vi "forceOutputState.vi"(8 "error in (no error)":errorcluster, 9 "calibratedValues":dbl[](array[numeric]), 10 "channel_addresses":string[](array[string]), 11 "niDAQmxAO in":refnum<class "niDAQmxAO.lvclass">) -> (0 "error out":errorcluster, 3 "niDAQmxAO out":refnum<class "niDAQmxAO.lvclass">)   [LabVIEW 2011, in "Hardware.lvlib" / "Channels.lvlib" / "niDAQmxAO.lvclass"]
uses:
  niDAQmxAO.lvclass
  <vilib>/DAQmx/write.llb/DAQmx Write (Analog DBL 1Chan 1Samp).vi
  <vilib>/DAQmx/write.llb/DAQmx Write (Analog 1D DBL NChan 1Samp).vi
  <vilib>/DAQmx/create/channels.llb/DAQmx Create Channel (AO-Voltage-Basic).vi
  <vilib>/DAQmx/miscellaneous.llb/DAQmx Fill In Error Info.vi
  AnalogOutput.lvclass
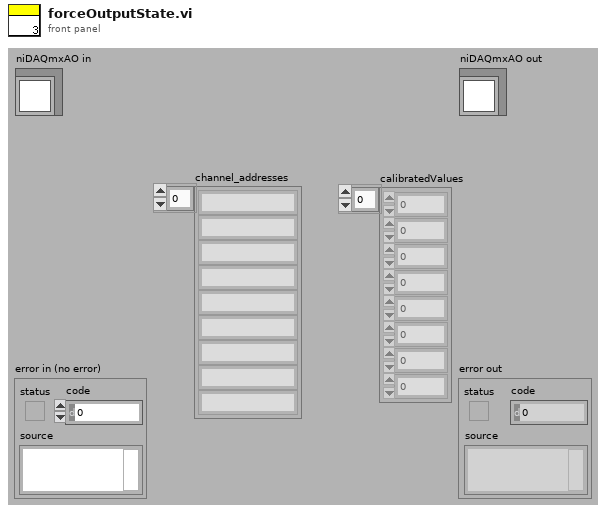
[diagram p1: front panel]
types:
  T1 = cluster{"channel_addresses":string[], "calibratedValues":dbl[]}
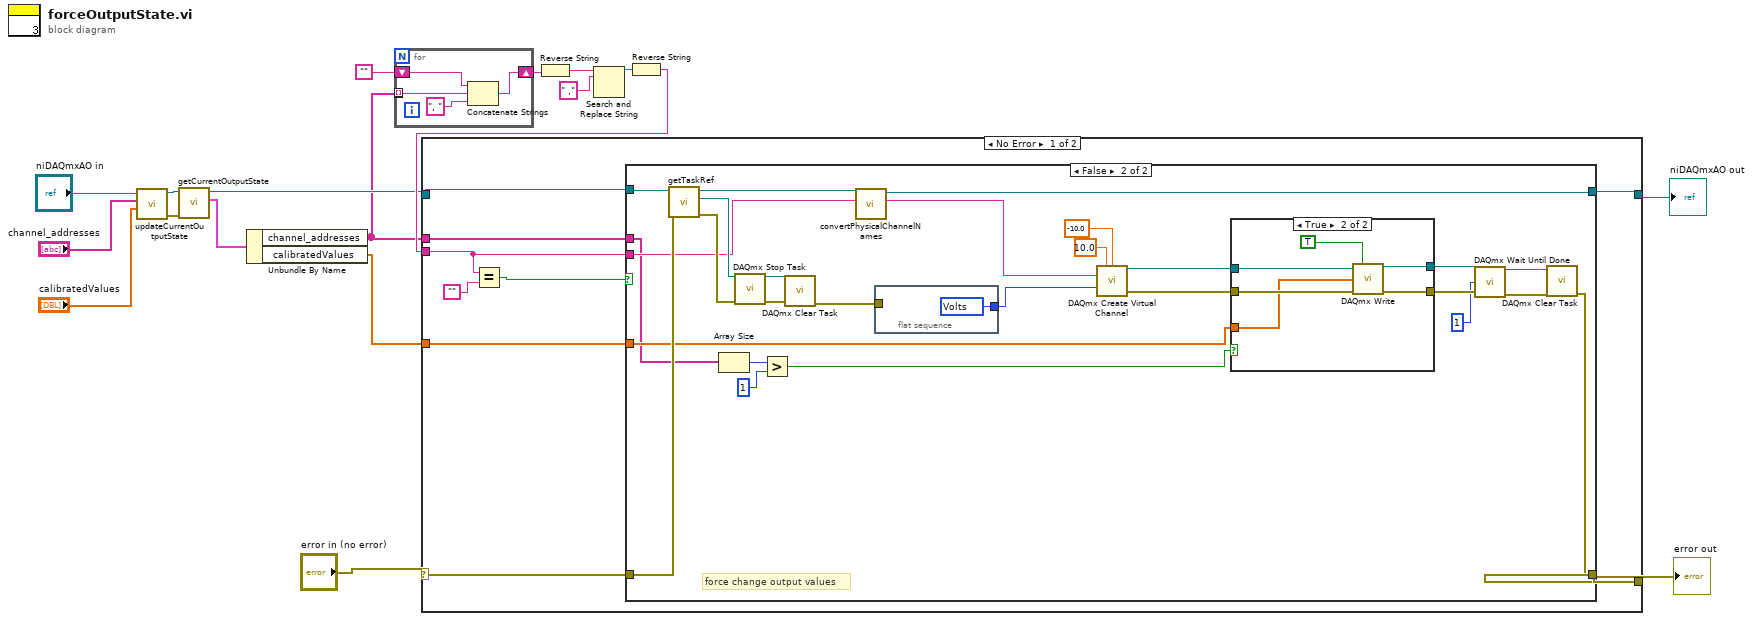
[diagram p0: block diagram]
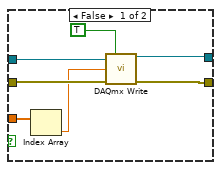
[diagram p3: hidden frame]
diagram:
  n1 = call "updateCurrentOutputState.vi"("calibratedValues"="calibratedValues", "channel_addresses"="channel_addresses", "AnalogOutput in"="niDAQmxAO in") -> ("error out"=w5:errorcluster, "AnalogOutput out"=w6:refnum<class "niDAQmxAO.lvclass">)  [unwired: 7 in]
  n2 = call "getCurrentOutputState.vi"("error in (no error)"=w5, "AnalogOutput.lvclass in"=w6) -> ("CurrentOutputState"=w4:T1, "AnalogOutput.lvclass out"=w3:refnum<class "niDAQmxAO.lvclass">)  [unwired: 7 in, 1 out]
  n3 = Unbundle By Name(w4) -> ("channel_addresses"=w1:string[], "calibratedValues"=w2:dbl[])
  n4 = for {
    tunnel: w1 -> [w21] mode=indexing
    tunnel: [w21] -> _ mode=indexing
    shift-right: [w19] -> w15
    shift-left: "" -> [w22]
    n5 = Concatenate Strings(w22, w21, ", ") -> (w19:string)
  }
  n6 = Reverse String(1:w15) -> (0:w14:string)
  n7 = Search and Replace String(input string=w14, search string=" ,") -> (result string=w12:string)  [unwired: 6 in, 3 out]
  n8 = Reverse String(1:w12) -> (0:w11:string)
  n9 = case shown="No Error" "error in (no error)" {
    selector: "error in (no error)" -> [w30 w75]
    tunnel: [w26 w76] -> w18
    tunnel: w3 -> [w31 w76]
    tunnel: w11 -> [w27 _]
    tunnel: [w25 w75] -> w10
    tunnel: w2 -> [w24 _]
    tunnel: w1 -> [w23 _]
    frame No Error {
      n10 = Equal?(x=w27, y="") -> (x = y?=w29:bool)
      n11 = case shown="False" w29 {
        tunnel: w27 -> [_ w44]
        tunnel: w31 -> [w33 w60]
        tunnel: [w33 w42] -> w26
        tunnel: w30 -> [w32 w59]
        tunnel: [w32 w50] -> w25
        tunnel: w24 -> [_ w38]
        tunnel: w23 -> [_ w37]
        frame True {
        }
        frame False {
          # "force change output values"
          n12 = call "getTaskRef.vi"("error in (no error)"=w59, "niDAQmxAO.lvclass in"=w60) -> ("error out"=w57:errorcluster, "DAQmx Task Ref"=w58:refnum<k21>, "niDAQmxAO.lvclass out"=w43:refnum<class "niDAQmxAO.lvclass">)  [unwired: 7 in]
          n13 = Array Size(array=w37) -> (size(s)=w36:i32)
          n14 = call <vilib>:"DAQmx Stop Task.vi"("task/channels in"=w58, "error in"=w57) -> ("task out"=w49:refnum<k21>, "error out"=w48:errorcluster)  [unwired: 12 in]
          n15 = Greater?(x=w36, y=1) -> (0:w34:bool)
          n16 = call <vilib>:"DAQmx Clear Task.vi"("task in"=w49, "error in"=w48) -> ("error out"=w47:errorcluster)  [unwired: 13 in]
          n17 = call "convertPhysicalChannelNames.vi"("PhysicalChannels"=w44, "niDAQmxAO.lvclass in"=w43) -> ("channel_names"=w41:string, "niDAQmxAO.lvclass out"=w42:refnum<class "niDAQmxAO.lvclass">)  [unwired: 7 in, 1 out]
          n18 = flat-sequence {
            tunnel: w47 -> [_]
            tunnel: [w74] -> w46
            frame #0 {
              w74 = 10348 items=["Volts"=10348, "From Custom Scale"=10065] ("units")
            }
          }
          n19 = call-poly <vilib>:"DAQmx Create Virtual Channel.vi"("maximum value"=10.0, "minimum value"=-10.0, "physical channels"=w41, "units"=w46) -> ("task out"=w40:refnum<k21>, "error out"=w39:errorcluster)  [unwired: 10 in]
          n20 = case shown="True" w34 {
            tunnel: [w63 w72] -> w54
            tunnel: [w64 w71] -> w53
            tunnel: w40 -> [w67 w70]
            tunnel: w39 -> [w65 w69]
            tunnel: w38 -> [w62 w68]
            frame False {
              n21 = Index Array(array=w62) -> (element=w61:dbl)  [unwired: 1 in]
              n22 = call-poly <vilib>:"DAQmx Write.vi"("task/channels in"=w67, "auto start"=TRUE, "data"=w61, "error in"=w65) -> ("task out"=w63:refnum<k21>, "error out"=w64:errorcluster)  [unwired: 9 in, 1 out]
            }
            frame True {
              n23 = call-poly <vilib>:"DAQmx Write.vi"("task/channels in"=w70, "auto start"=TRUE, "data"=w68, "error in"=w69) -> ("task out"=w72:refnum<k21>, "error out"=w71:errorcluster)  [unwired: 9 in, 1 out]
            }
          }
          n24 = call <vilib>:"DAQmx Wait Until Done.vi"("task/channels in"=w54, "timeout (sec)"=1, "error in"=w53) -> ("task out"=w52:refnum<k21>, "error out"=w51:errorcluster)  [unwired: 11 in]
          n25 = call <vilib>:"DAQmx Clear Task.vi"("task in"=w52, "error in"=w51) -> ("error out"=w50:errorcluster)  [unwired: 13 in]
        }
      }
    }
    frame Error {
    }
  }
  "error out" <- w10
  "niDAQmxAO out" <- w18
